vi "Current_Calib_Filenames.vi"(3 "Calib Filename":path[](array[path]), 4 "Channel ID input":string[](array[string]), 5 "Mode":T1) -> (0 "Calib Filename Out":path[](array[path]), 1 "Channel ID Output":string[](array[string]), 2 "Ch-CalPathArray":cluster{"String":string, "File Path":path}[](array[cluster]))   [LabVIEW 2021]
uses:
  Controls/App_Global.ctl
  File/Setup_Filetype.ctl
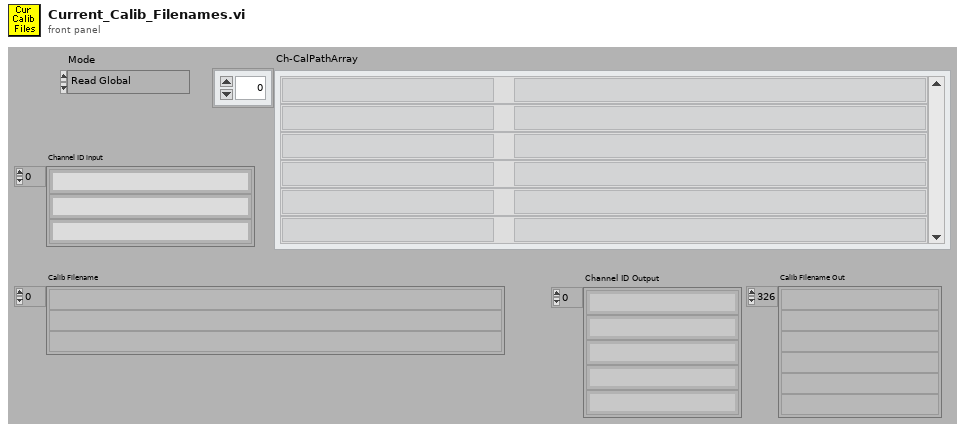
[diagram p1: front panel]
types:
  T1 = typedef "App_Global.ctl" = enum16{"Read Global", "Write to Global", "Initialise Array"}
  T2 = typedef "Setup_Filetype.ctl" = enum16{"Measurement Setups", "Calibration Setups", "General", "Results File Plotter Setups", "Speed Calib Tweaks"}
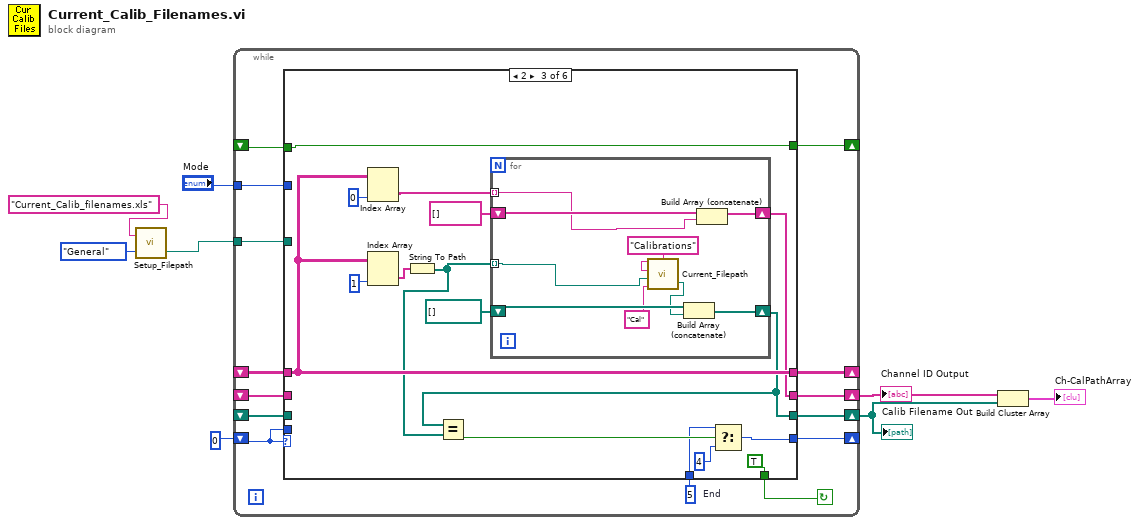
[diagram p0: block diagram]
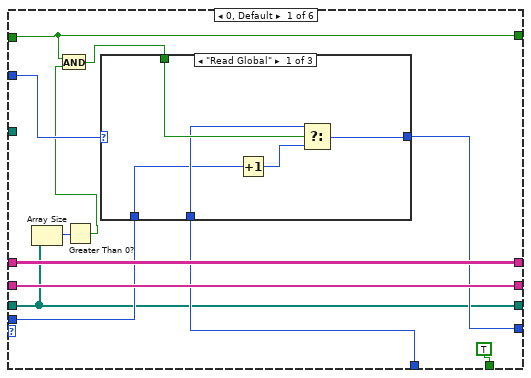
[diagram p2: hidden frame]
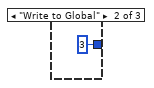
[diagram p3: hidden frame]
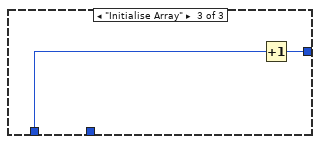
[diagram p4: hidden frame]
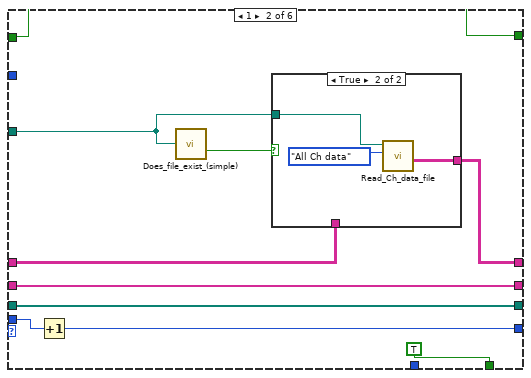
[diagram p5: hidden frame]
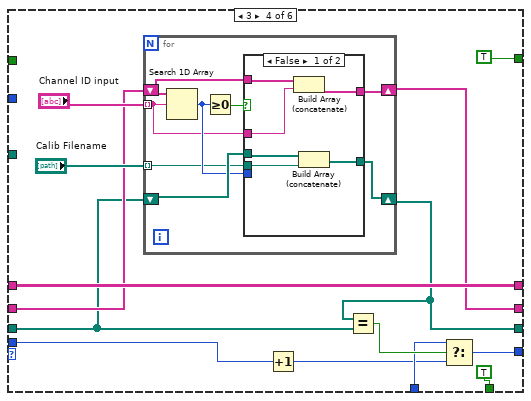
[diagram p7: hidden frame]
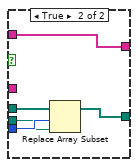
[diagram p8: hidden frame]
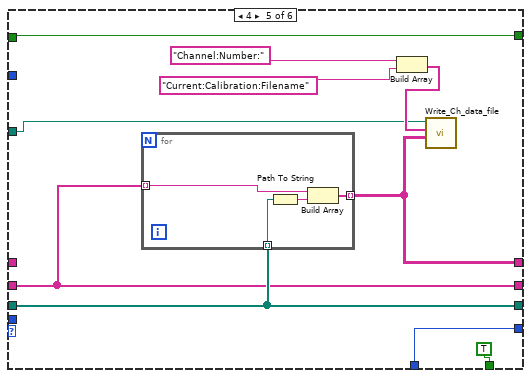
[diagram p9: hidden frame]
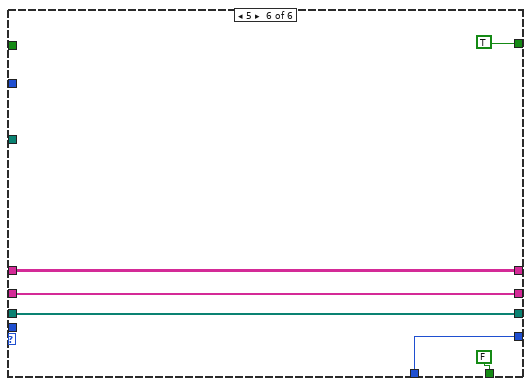
[diagram p10: hidden frame]
diagram:
  n1 = call "Setup_Filepath.vi"("Setup File Type"=Setup_Filetype."General", "Filename in"="Current_Calib_filenames.xls" ("Substring")) -> ("Filename Out"=w5:path)  [unwired: 1 out]
  n2 = while {
    shift-left: _ -> [w11]
    shift-right: [w13] -> w2
    shift-left: _ -> [w12]
    shift-right: [w14] -> w3
    tunnel: "Mode" -> [w18]
    shift-left: 0 -> [w19]
    shift-right: [w20] -> _
    shift-left: _ -> [w15]
    shift-right: [w16] -> _
    shift-left: _ -> [w22]
    shift-right: [w17] -> _
    tunnel: w5 -> [w9]
    stop <- w21 continue-if-true
    w10 = 5  # End
    n3 = case shown="2" w19 {
      tunnel: w22 -> [w25 w49 w68 _ w124 _]
      tunnel: [TRUE TRUE TRUE TRUE TRUE FALSE] -> w21
      tunnel: [w28 w50 w60 w82 w123 w130] -> w20
      tunnel: w19 -> [w29 w51 _ w84 _ _]
      tunnel: w18 -> [w31 _ _ _ _ _]
      tunnel: [w25 w49 w68 TRUE w124 TRUE] -> w17
      tunnel: [w33 w47 w67 w94 w116 w133] -> w16
      tunnel: w15 -> [w33 w46 w67 w94 _ w133]
      tunnel: [w34 w45 w65 w89 w117 w132] -> w14
      tunnel: [w27 w44 w64 w88 w118 w131] -> w13
      tunnel: w12 -> [w34 w45 _ w90 w117 w132]
      tunnel: w11 -> [w27 w44 _ w87 w118 w131]
      tunnel: w10 -> [w30 _ w61 w85 w123 w130]
      tunnel: w9 -> [_ w43 _ _ w115 _]
      frame 0, Default {
        n4 = Array Size(array=w27) -> (size(s)=w26:i32)
        n5 = Greater Than 0?(x=w26) -> (x > 0?=w24:bool)
        n6 = And(x=w25, y=w24) -> (x .and. y?=w23:bool)
        n7 = case shown="\"Read Global\"" w31 {
          tunnel: w23 -> [w39 _ _]
          tunnel: w30 -> [w38 _ _]
          tunnel: w29 -> [w36 _ w42]
          tunnel: [w35 3 ("End") w41] -> w28
          frame "Read Global" {
            n8 = Increment(x=w36) -> (x+1=w37:i32)
            n9 = Select(t=w38, s=w39, f=w37) -> (s? t:f=w35:i32)
          }
          frame "Write to Global" {
          }
          frame "Initialise Array" {
            n10 = Increment(x=w42) -> (x+1=w41:i32)
          }
        }
      }
      frame 1 {
        n11 = Increment(x=w51) -> (x+1=w50:i32)
        n12 = call "Does_file_exist_(simple).vi"("Pathname"=w43) -> ("exists?"=w48:bool)
        n13 = case shown="True" w48 {
          tunnel: w43 -> [_ w55]
          tunnel: [w53 w54] -> w47
          tunnel: w46 -> [w53 _]
          frame False {
          }
          frame True {
            n14 = call "Read_Ch_data_file.vi"("Output"=enum16{"All Ch data", "The last few rows"}."All Ch data", "Filename"=w55) -> ("Channel Values"=w54:string[][])  [unwired: 3 in, 4 out]
          }
        }
      }
      frame 2 {
        n15 = Index Array(array=w67, index (col)=0 ("Index")) -> (element=w58:string[])  [unwired: 1 in]
        n16 = Index Array(array=w67, index (col)=1 ("Index")) -> (element=w69:string[])  [unwired: 1 in]
        n17 = String To Path(string=w69) -> (path=w63:path[])
        n18 = for {
          shift-right: [w80] -> w65
          shift-right: [w77] -> w64
          shift-left: path[] [] -> [w78]
          tunnel: w63 -> [w76] mode=indexing
          shift-left: string[] [] -> [w81]
          tunnel: w58 -> [w79] mode=indexing
          n19 = call "Current_Filepath.vi"("Short_Name"="Cal", "Filename in"=w76, "Data Type"="Calibrations") -> ("Filename Out"=w74:path)  [unwired: 1 in, 1 out]
          n20 = Build Array (concatenate)(w78, w74) -> (w77:path[])
          n21 = Build Array (concatenate)(w81, w79) -> (w80:string[])
        }
        n22 = Equal?(x=w64, y=w63) -> (x = y?=w62:bool)
        n23 = Select(t=w61, s=w62, f=4) -> (s? t:f=w60:i32)
      }
      frame 3 {
        n24 = for {
          tunnel: "Channel ID input" -> [w96] mode=indexing
          shift-right: [w99] -> w88
          shift-left: w87 -> [w102]
          tunnel: "Calib Filename" -> [w100] mode=indexing
          shift-right: [w98] -> w89
          shift-left: w90 -> [w97]
          n25 = Search 1D Array(1D array=w97, element=w96) -> (index of element=w101:i32)  [unwired: 1 out]
          n26 = Greater Or Equal To 0?(x=w101) -> (x >= 0?=w103:bool)
          n27 = case shown="False" w103 {
            tunnel: w102 -> [w106 w114]
            tunnel: w101 -> [_ w113]
            tunnel: w100 -> [w105 w112]
            tunnel: [w104 w111] -> w99
            tunnel: [w107 w110] -> w98
            tunnel: w97 -> [w109 w110]
            tunnel: w96 -> [w108 _]
            frame False {
              n28 = Build Array (concatenate)(w109, w108) -> (w107:string[])
              n29 = Build Array (concatenate)(w106, w105) -> (w104:path[])
            }
            frame True {
              n30 = Replace Array Subset(array=w114, new element=w112, index=w113) -> (w111:path[])
            }
          }
        }
        n31 = Increment(x=w84) -> (x+1=w83:i32)
        n32 = Equal?(x=w88, y=w87) -> (x = y?=w86:bool)
        n33 = Select(t=w85, s=w86, f=w83) -> (s? t:f=w82:i32)
      }
      frame 4 {
        n34 = for {
          tunnel: w118 -> [w128] mode=indexing
          tunnel: w117 -> [w125] mode=indexing
          tunnel: [w127] -> w116 mode=indexing
          n35 = Path To String(path=w128) -> (string=w126:string)
          n36 = Build Array(w125, w126) -> (w127:string[])
        }
        n37 = Build Array("Channel:Number:", "Current:Calibration:Filename") -> (w119:string[])
        n38 = call "Write_Ch_data_file.vi"("Channel Values"=w116, "Channel names"=w119, "Filename"=w115) -> ()  [unwired: 5 in, 4 out]
      }
      frame 5 {
      }
    }
  }
  "Channel ID Output" <- w3
  "Calib Filename Out" <- w2
  n39 = Build Cluster Array(w3, w2) -> (→"Ch-CalPathArray":cluster{"Ch No":string, "Ch No":path}[])
